vi "SwerveKinematics.vi"(0 "Joystick X":dbl(slide) scale=-1.0..1.0, 5 "Joystick Y":dbl(slide) scale=1.0..-1.0, 7 "Joystick Rotation":dbl(slide) scale=1.0..-1.0, 9 "Cx (in)":dbl, 11 "Cy (in)":dbl) -> (1 "Module 0 Angle (deg)":dbl(knob) scale=180.0..-180.0 scale format="%#_6f", 3 "Module 1 Angle (deg)":dbl(knob) scale=180.0..-180.0 scale format="%#_6f", 4 "Module 0 Velocity Command (ul)":dbl(slide) scale=0.0..1.0 scale format="%.2f", 6 "Module 1 Velocity Command (ul)":dbl(slide) scale=0.0..1.0 scale format="%.2f", 10 "Module 2 Velocity Command (ul)":dbl(slide) scale=0.0..1.0 scale format="%.2f", 12 "Module 3 Angle (deg)":dbl(knob) scale=180.0..-180.0 scale format="%#_6f", 14 "Module 2 Angle (deg)":dbl(knob) scale=180.0..-180.0 scale format="%#_6f", 15 "Module 3 Velocity Command (ul)":dbl(slide) scale=0.0..1.0 scale format="%.2f")   [LabVIEW 2019]
doc: "Performs the kinematics for a rectangular four wheel swerve robot with a selectable center of rotation. Swerve module #0 is located in the front right corner and the modules increment in the counter-clockwise direction."
panel:
  in  "Robot_Width (in)":dbl=28.0
  in  "Robot_Length (in)":dbl=28.0
  # "\"Front\" of Robot"
  # "M1"
  # "M0"
  # "Left Thumbstick"
  # "Right Thumbstick"
  # "X"
  # "Y"
  # "(0,0)"
  # "+CCW"
  # "M2"
  # "M3"
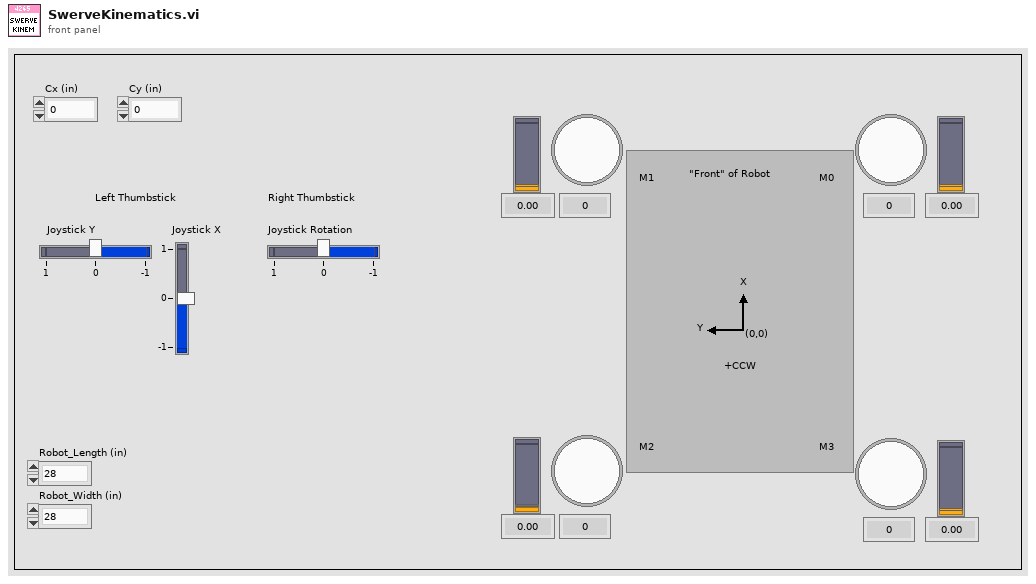
[diagram p1: front panel]
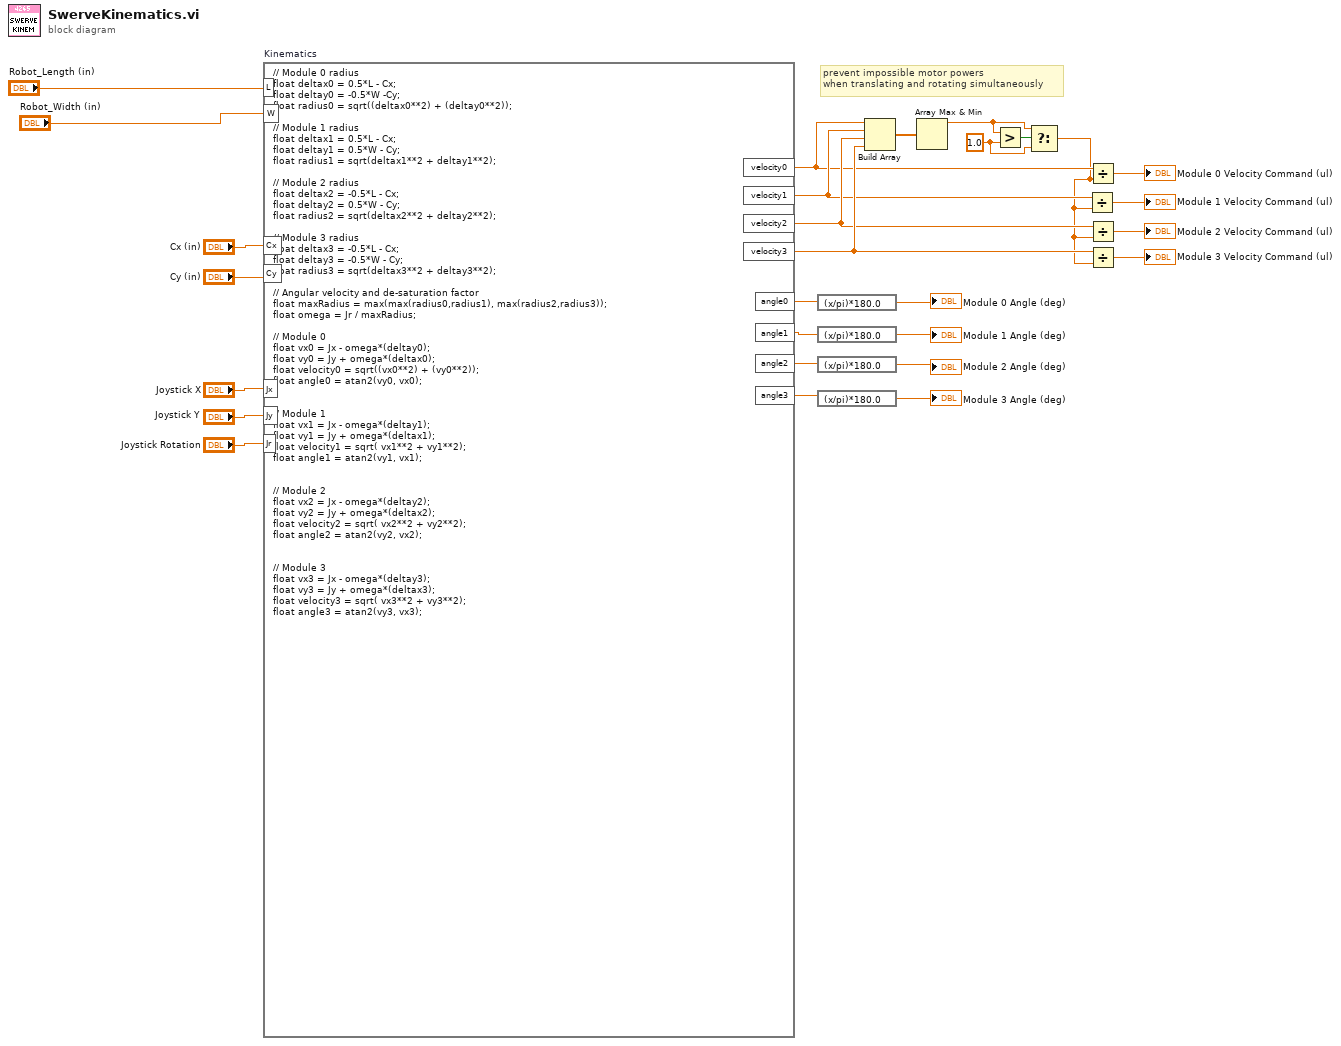
[diagram p0: block diagram]
diagram:
  w20 = 1.0 ("y")
  # "prevent impossible motor powers\nwhen translating and rotating simultaneously"
  n1 = formula code="// Module 0 radius\nfloat deltax0 = 0.5*L - Cx;\nfloat deltay0 = -0.5*W -Cy; \nfloat radius0 = sqrt((deltax0**2) + (deltay0**2));\n\n// Module 1 radius\nfloat deltax1 = 0.5*L - Cx;\nfloat deltay1 = 0.5*W - Cy;\nfloat radius1 = sqrt(deltax1**2 + deltay1**2);\n\n// Module 2 radius\nfloat deltax2 = -0.5*L - Cx;\nfloat deltay2 = 0.5*W - Cy;\nfloat radius2 = sqrt(deltax2**2 + deltay2**2);\n\n// Module 3 radius\nfloat deltax3 = -0.5*L - Cx;\nfloat deltay3 = -0.5*W - Cy;\nfloat radius3 = sqrt(deltax3**2 + deltay3**2);\n\n// Angular velocity and de-saturation factor\nfloat maxRadius = max(max(radius0,radius1), max(radius2,radius3));\nfloat omega = Jr / maxRadius;\n\n// Module 0\nfloat vx0 = Jx - omega*(deltay0);\nfloat vy0 = Jy + omega*(deltax0);\nfloat velocity0 = sqrt((vx0**2) + (vy0**2));\nfloat angle0 = atan2(vy0, vx0);\n\n\n// Module 1\nfloat vx1 = Jx - omega*(deltay1);\nfloat vy1 = Jy + omega*(deltax1);\nfloat velocity1 = sqrt( vx1**2 + vy1**2);\nfloat angle1 = atan2(vy1, vx1);\n\n\n// Module 2\nfloat vx2 = Jx - omega*(deltay2);\nfloat vy2 = Jy + omega*(deltax2);\nfloat velocity2 = sqrt( vx2**2 + vy2**2);\nfloat angle2 = atan2(vy2, vx2);\n\n\n// Module 3\nfloat vx3 = Jx - omega*(deltay3);\nfloat vy3 = Jy + omega*(deltax3);\nfloat velocity3 = sqrt( vx3**2 + vy3**2);\nfloat angle3 = atan2(vy3, vx3);" "Kinematics"("L"="Robot_Length (in)", "W"="Robot_Width (in)", "Cx"="Cx (in)", "Cy"="Cy (in)", "Jr"="Joystick Rotation", "Jx"="Joystick X", "Jy"="Joystick Y") -> ("velocity0"=w14:dbl, "angle0"=w26:dbl, "angle1"=w24:dbl, "angle2"=w23:dbl, "angle3"=w22:dbl, "velocity1"=w15:dbl, "velocity2"=w16:dbl, "velocity3"=w17:dbl)
  n2 = expression code="(x/pi)*180.0" ("radians to degrees")(w26) -> (→"Module 0 Angle (deg)":dbl)
  n3 = expression code="(x/pi)*180.0" ("radians to degrees")(w24) -> (→"Module 1 Angle (deg)":dbl)
  n4 = expression code="(x/pi)*180.0" ("radians to degrees")(w23) -> (→"Module 2 Angle (deg)":dbl)
  n5 = expression code="(x/pi)*180.0" ("radians to degrees")(w22) -> (→"Module 3 Angle (deg)":dbl)
  n6 = Build Array(w14, w15, w16, w17) -> (w18:dbl[])
  n7 = Array Max & Min(array=w18) -> (max value=w19:dbl)  [unwired: 3 out]
  n8 = Greater?(x=w19, y=w20) -> (0:w21:bool)
  n9 = Select(t=w19, s=w21, f=w20) -> (s? t:f=w5:dbl)
  n10 = Divide(x=w15, y=w5) -> (x/y=→"Module 1 Velocity Command (ul)":dbl)
  n11 = Divide(x=w14, y=w5) -> (x/y=→"Module 0 Velocity Command (ul)":dbl)
  n12 = Divide(x=w16, y=w5) -> (x/y=→"Module 2 Velocity Command (ul)":dbl)
  n13 = Divide(x=w17, y=w5) -> (x/y=→"Module 3 Velocity Command (ul)":dbl)
